vi "版本号(子VI).vi"(9 "数字 3":u16, 10 "数字 2":u16, 11 "数字":u16) -> (3 "结果字符串":string)   [LabVIEW 2016, in "德润DR803L超标留样.lvlib"]
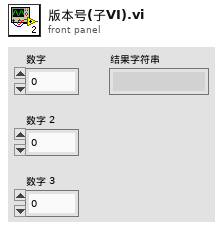
[diagram p1: front panel]
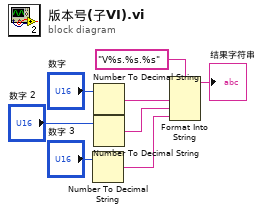
[diagram p0: block diagram]
diagram:
  n1 = Number To Decimal String(number="数字 3") -> (decimal integer string=w4:string)  [unwired: 1 in]
  n2 = Number To Decimal String(number="数字") -> (decimal integer string=w2:string)  [unwired: 1 in]
  n3 = Number To Decimal String(number="数字 2") -> (decimal integer string=w3:string)  [unwired: 1 in]
  n4 = Format Into String(format string="V%s.%s.%s" ("格式字符串"), w2, w3, w4) -> (resulting string=→"结果字符串":string)  [unwired: 2 in, 1 out]
